vi "Dashboard Main.vi"() -> ()   [LabVIEW 2018]
uses:
  <vilib>/Utility/miscctls.llb/LVBoundsTypeDef.ctl
  <vilib>/Utility/miscctls.llb/LVRowAndColumnTypeDef.ctl
  <vilib>/event_ctls.llb/eventvkey.ctl
  <vilib>/Rock Robotics/Network Tables/NT Read Numeric Array.vi
  <vilib>/Rock Robotics/Network Tables/NT Write Boolean.vi
  <vilib>/Rock Robotics/WPI/Dashboard/WPI_DashboardLogging Global.vi
panel:
  in  "Camera Settings Right":T1={"Frame Rate"=30, "Compression"=30, "Size"=1, "DB Camera Config"=FALSE} {"Frame Rate" scale=1.0..30.0; "Compression" scale=100.0..-1.0; "Size" items=["640x480", "320x240", "160x120"]}
  in  "Camera Name Right":string(combo)="No Camera Selection"
  out "Camera Perf":string
  in  "Camera Settings":T1={"Frame Rate"=30, "Compression"=30, "Size"=1, "DB Camera Config"=FALSE} {"Frame Rate" scale=1.0..30.0; "Compression" scale=100.0..-1.0; "Size" items=["640x480", "320x240", "160x120"]}
  in  "TCP":refnum<k5>
  in  "Rec Mode":enum32{"Stop", "Record", "Playback"}(radio)
  out "Robot IP":string
  out "Image Message":string="Timeout in Camera Communications"
  in  "Dashboard Tab":T2(tab)
  in  "Select Auto":string(combo)="Select Autonomous ..."
  out "NT Connection":bool
  out "MotorChart R":cluster{"Numeric":dbl, "Numeric":dbl}(graph)
  out "MotorChart L":cluster{"Numeric":dbl, "Numeric":dbl}(graph)
  out "MotorSliders R":cluster{"MotorSlide1":dbl, "MotorSlide2":dbl} {"MotorSlide2" scale=-1.0..1.0 scale format="%#_2e"; "MotorSlide1" scale=-1.0..1.0 scale format="%#_2e"}
  out "MotorSliders L":cluster{"MotorSlide1":dbl, "MotorSlide2":dbl} {"MotorSlide2" scale=-1.0..1.0 scale format="%#_2e"; "MotorSlide1" scale=-1.0..1.0 scale format="%#_2e"}
  out "Gyro_defualt":dbl(knob) scale=0.0..360.0
  out "JS1 Z":dbl(slide) scale=-1.0..1.0 scale format="%#_2e"
  out "JS1 Graph":cluster{"X":dbl, "Y":dbl}[](graph)
  out "JS1 Buttons":T3
  out "JS2 Z":dbl(slide) scale=-1.0..1.0 scale format="%#_2e"
  out "JS2 Graph":cluster{"X":dbl, "Y":dbl}[](graph)
  out "JS2 Buttons":T3
  out "Mode":T4(ring)=enum."Auto Disabled"
  out "Right Camera Perf":cluster{"Bandwidth (Mbps)":dbl, "FPS":dbl}
  out "Camera Image Right":T5(plugin-control)
  in  "DB/String 9":string
  in  "DB/String 8":string
  in  "DB/String 7":string
  in  "DB/String 6":string
  in  "DB/String 5":string
  in  "DB/String 4":string
  in  "DB/String 3":string
  in  "DB/String 2":string
  in  "DB/String 1":string
  in  "DB/String 0":string
  in  "DB/Slider 0":dbl(slide) scale=0.0..5.0
  in  "DB/Slider 1":dbl(slide) scale=0.0..5.0
  in  "DB/Slider 2":dbl(slide) scale=0.0..5.0
  in  "DB/Slider 3":dbl(slide) scale=0.0..5.0
  out "DB/LED 3":bool
  out "DB/LED 2":bool
  out "DB/LED 1":bool
  out "DB/LED 0":bool
  in  "DB/Button 3":bool
  in  "DB/Button 2":bool
  in  "DB/Button 1":bool
  in  "DB/Button 0":bool caption="New Name"
  out "Gyro":dbl
  out "Cargo 0":bool
  out "Cargo 3":bool
  out "Cargo 1":bool
  out "Cargo 2":bool
  out "Hatch 2":bool
  out "Hatch 0":bool
  out "Hatch 1":bool
  out "Elevator Position":dbl(slide) scale=0.0..20000.0
  out "Cargo Drop":bool
  out "Cargo Pick Up":bool
  out "Carry":bool
  out "Hatch":bool
  in  "Calibrate?":bool
  out "PickUp/DropOff":string
  out "SwerveMode":string
  in  "Test Slider":dbl(slide) scale=0.0..100.0 scale format="%#_3g"
  in  "On/Off":bool caption="Solenoid"
  in  "Test Name":u16(ring) items=["Select the test to run..."]
  in  "Test Tree":string(tree)
  in  "Motor":cluster{"Value":dbl, "Enable":bool} {"Value" scale=-1.0..1.0 scale format="%#_3g"}
  out "Progress":T6 {"Test Progress" scale=0.0..100.0}
  in  "Rev/Fwd":cluster{"Forward":bool, "Reverse":bool}
  in  "Test Ring":u16(ring) items=["Monochrome", "Color"]
  out "Cmd Status":string
  in  "Execute Command":bool
  in  "Command Params":string[][](table)
  in  "Command Selection":i32(listbox)
  in  "CheckList":i32(listbox)
  out "Tree":string(tree)
  out "Camera Image":T5(plugin-control)
  out "Background":bool
  in  "Camera Name":string(combo)="No Camera Selection"
  # "HW"
  # "HW"
  # "Joysticks"
  # "Drive Motors"
  # "Front"
  # "Right"
  # "Left"
  # "Back"
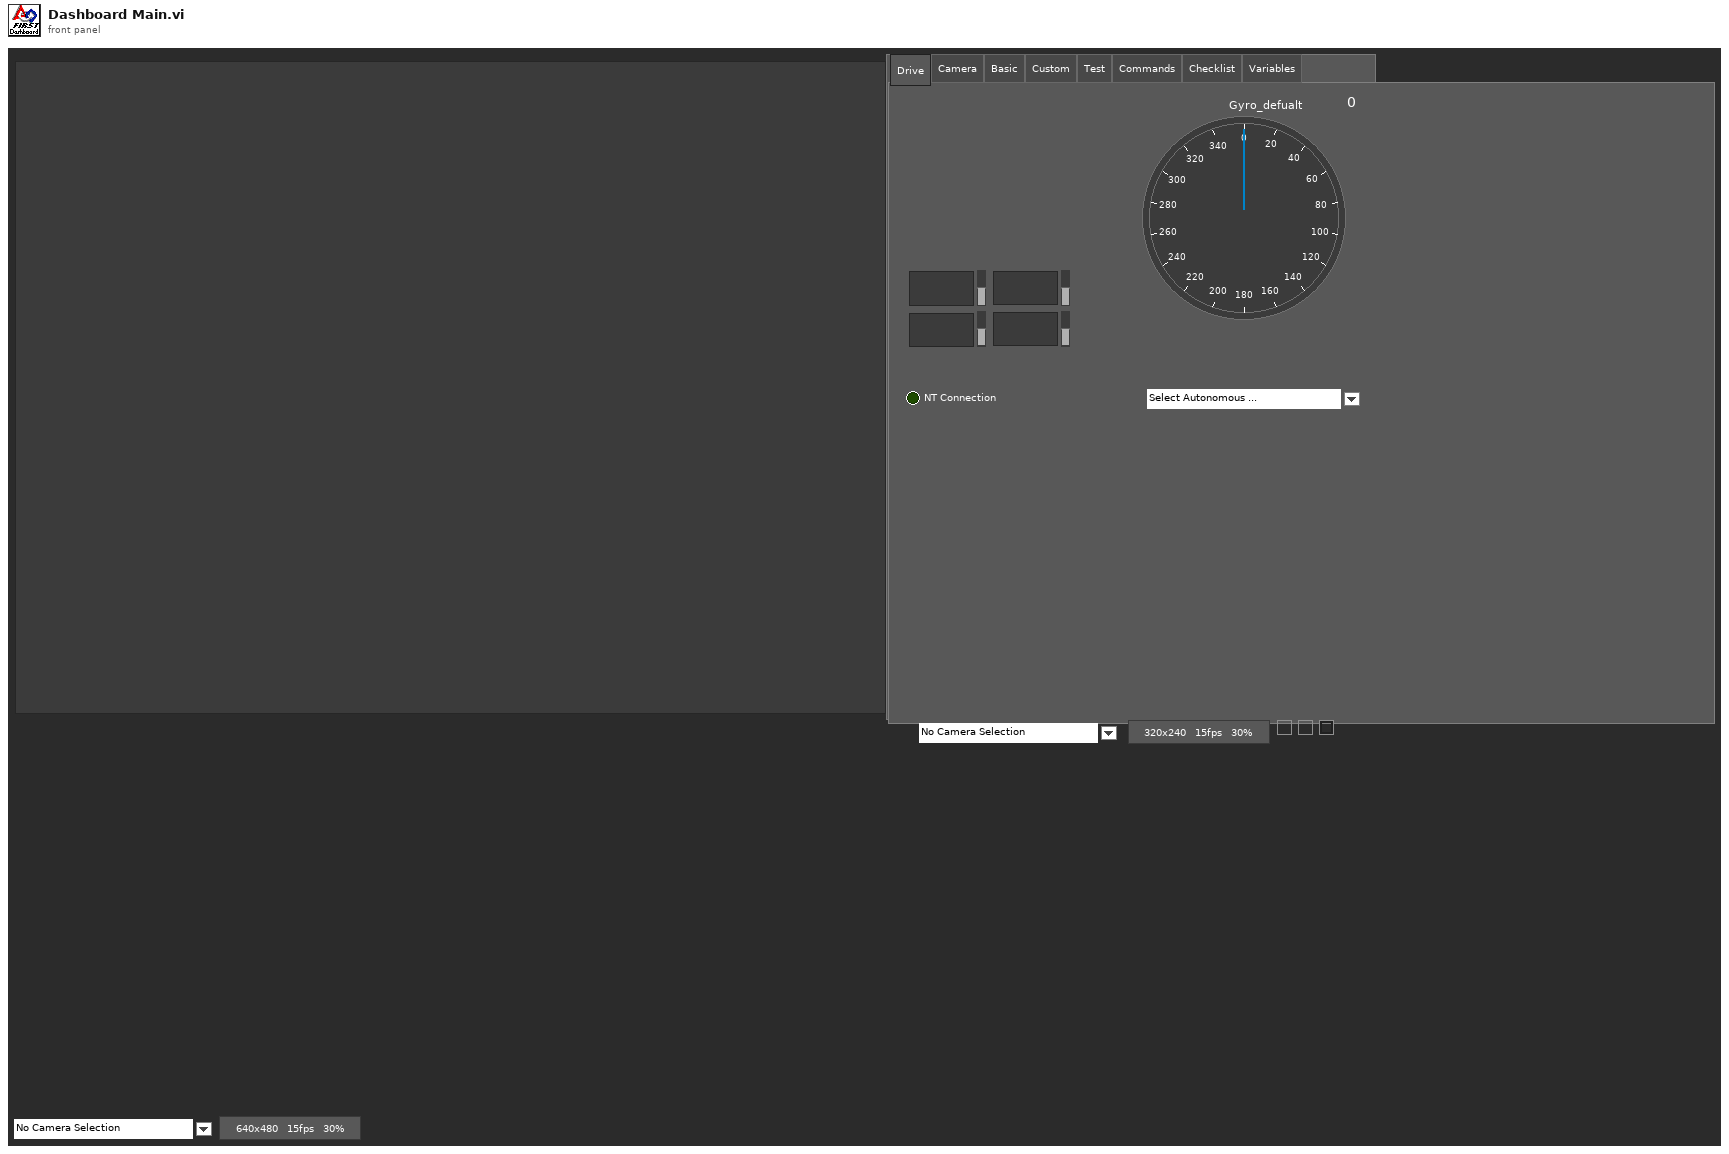
[diagram p1: front panel]
types:
  T1 = cluster{"Frame Rate":i32, "Compression":i32, "Size":u16, "DB Camera Config":bool}
  T2 = enum32{"Drive", "Camera", "Basic", "Custom", "Test", "Commands", "Checklist", "Variables"}
  T3 = cluster{bool, bool, bool, bool, bool, bool, bool, bool, bool, bool, bool, bool}
  T4 = enum8{"Tele-Op Disabled", "Tele-Op Enabled", "Auto Disabled", "Auto Enabled", "Test Disabled", "Test Enabled", "Disconnected", "No Code", "E-Stop"}
  T5 = typedef "IMAQ Image.ctl" = refnum<image>
  T6 = cluster{"Test Progress":u8, "Test Progress Text":string}
  T7 = typedef "LVBoundsTypeDef.ctl" = cluster{"Width":u32, "Height":u32}
  T8 = cluster{"Save Path":path, "Interval (s)":dbl, "Keep":i32}
  T9 = typedef "Image Type" = u32
  T10 = cluster{"IDs":cluster{"RPC field ID":u16, "Unique ID":u16}, "String":string}
  T11 = cluster{"Error Strings":string, "Disable Counts":cluster{u16, u16}, "Rail Faults":cluster{u16, u16, u16}, "Robot IP":string, "DB Mode":u8, "Event Info":cluster{"Name":string, "Type":u8, "Number":u16, "Replay":u8}}
  T12 = cluster{"Storage":cluster{"Disk Free":u64, "RAM Block":u32, "RAM free":u32}, "CPU Utilization":cluster{"CPU % ISR":sgl, "CPU % Time Crit":sgl, "CPU % Timed Str":sgl, "CPU % High":sgl, "CPU % Above":sgl, "CPU % Normal":sgl, "CPU % Low":sgl}, "CAN":cluster{"% Bus Utilization":sgl, "Bus Off Cnt":u32, "TX_FIFO Full Cnt":u32, "Receive Error Cnt":u8, "Transmit Error Cnt":u8}, "HID":cluster{"HID Outputs":u32, "Rumble Low":u16, "Rumble High":u16}[]}
  T13 = cluster{"Status bits":cluster{"Test Mode":bool, "Autonomous":bool, "Enabled":bool, "Code Start":bool, "Brownout":bool, "Reserved 2":bool, "Reserved 3":bool, "E-Stop":bool}, "Code Trace":cluster{"Disabled":bool, "TeleOp":bool, "Auto":bool, "Test":bool}, "Controller Type":enum16{"unknown", "cRIO", "roboRio"}, "Code?":enum16{"unknown", "noCode", "code"}, "Battery V":dbl}
  T14 = cluster{"Control Bits":cluster{"TestMode":bool, "Autonomous":bool, "Enabled":bool, "FMS Present":bool, bool, bool, bool, "E-Stop":bool}, "Team Station ":u8, "Countdown":sgl, "Joystick Values":cluster{"Axes":dbl[], "Buttons":bool[], "POVs":i16[]}[]}
  T15 = cluster{"Axes":dbl[], "Buttons":bool[], "POVs":i16[]}[]
  T16 = cluster{"Axes":dbl[], "Buttons":bool[], "POVs":i16[]}
  T17 = cluster{"Buttons[0]":bool, "Buttons[1]":bool, "Buttons[2]":bool, "Buttons[3]":bool, "Buttons[4]":bool, "Buttons[5]":bool, "Buttons[6]":bool, "Buttons[7]":bool, "Buttons[8]":bool, "Buttons[9]":bool, "Buttons[10]":bool, "Buttons[11]":bool}
  T18 = cluster{"Camera Image":refnum<vi>, "Dashboard Tab":refnum<vi>, "Background":refnum<vi>, "Rec Mode":refnum<vi>, "Test Slider":refnum<vi>, "On/Off ":refnum<vi>, "Test Ring":refnum<vi>, "Rev/Fwd":refnum<vi>, "Test Name":refnum<vi>, "Motor":refnum<vi>, "Progress":refnum<vi>, "CheckList":refnum<vi>, "Tree":refnum<vi>, "Test Tree":refnum<vi>, "Command Params":refnum<vi>, "Command Selection":refnum<vi>, "Execute Command":refnum<vi>, "Cmd Status":refnum<vi>, "Camera Settings":refnum<vi>, "Camera Name":refnum<vi>, "Camera Perf":refnum<vi>, "Camera Settings Right":refnum<vi>, "Camera Name Right":refnum<vi>, "Camera Image Right":refnum<vi>}
  T19 = cluster{"Global Rectangle":i32[], "Contours":cluster{"Contour Type":u32, "ROI Type":u32, "Points":i32[]}[]}
  T20 = cluster{"Camera Name":string, string, "Saved DB Images Info":cluster{"Save Path":path, "Interval (s)":dbl, "Keep":i32}}
  T21 = cluster{"Camera Name Right":string, string, "Saved DB Images Info":cluster{"Save Path":path, "Interval (s)":dbl, "Keep":i32}}
  T22 = cluster{"Operation":enum16{"Update", "Clear"}, "Color Box":u32}[]
  T23 = typedef "eventvkey.ctl" = enum16{"ASCII", "Enter", "Return", "Shift", "Ctrl", "Alt", "Cmd", "Opt", "Caps", "NumLock", "Clear", "Break", "Up", "Down", "Left", "Right", "Insert", "Delete", "Home", "End", "PageUp", "PageDown", "Escape", "Help", "Pause", "ScrollLock", "F1", "F2", "F3", "F4", "F5", "F6", "F7", "F8", "F9", "F10", "F11", "F12", "F13", "F14", "F15", "F16", "F17", "F18", "F19", "F20", "F21", "F22", "F23", "F24", "Play", "VolumeUp", "VolumeDown", "Mute", "Two Byte Char"}
  T24 = cluster{"Image Size":bool, "Image Type":bool, "Pixel Value":bool, "ROI Information":bool, "Zoom Factor":bool}
  T25 = cluster{"Operation":enum16{"Update", "Clear"}, "Color Box":u32}
  T26 = typedef "LVRowAndColumnTypeDef.ctl" = cluster{"Row":i32, "Column":i32}
  T27 = cluster{"Shift":bool, "Ctrl":bool, "Alt":bool, "Cmd":bool, "Opt":bool}
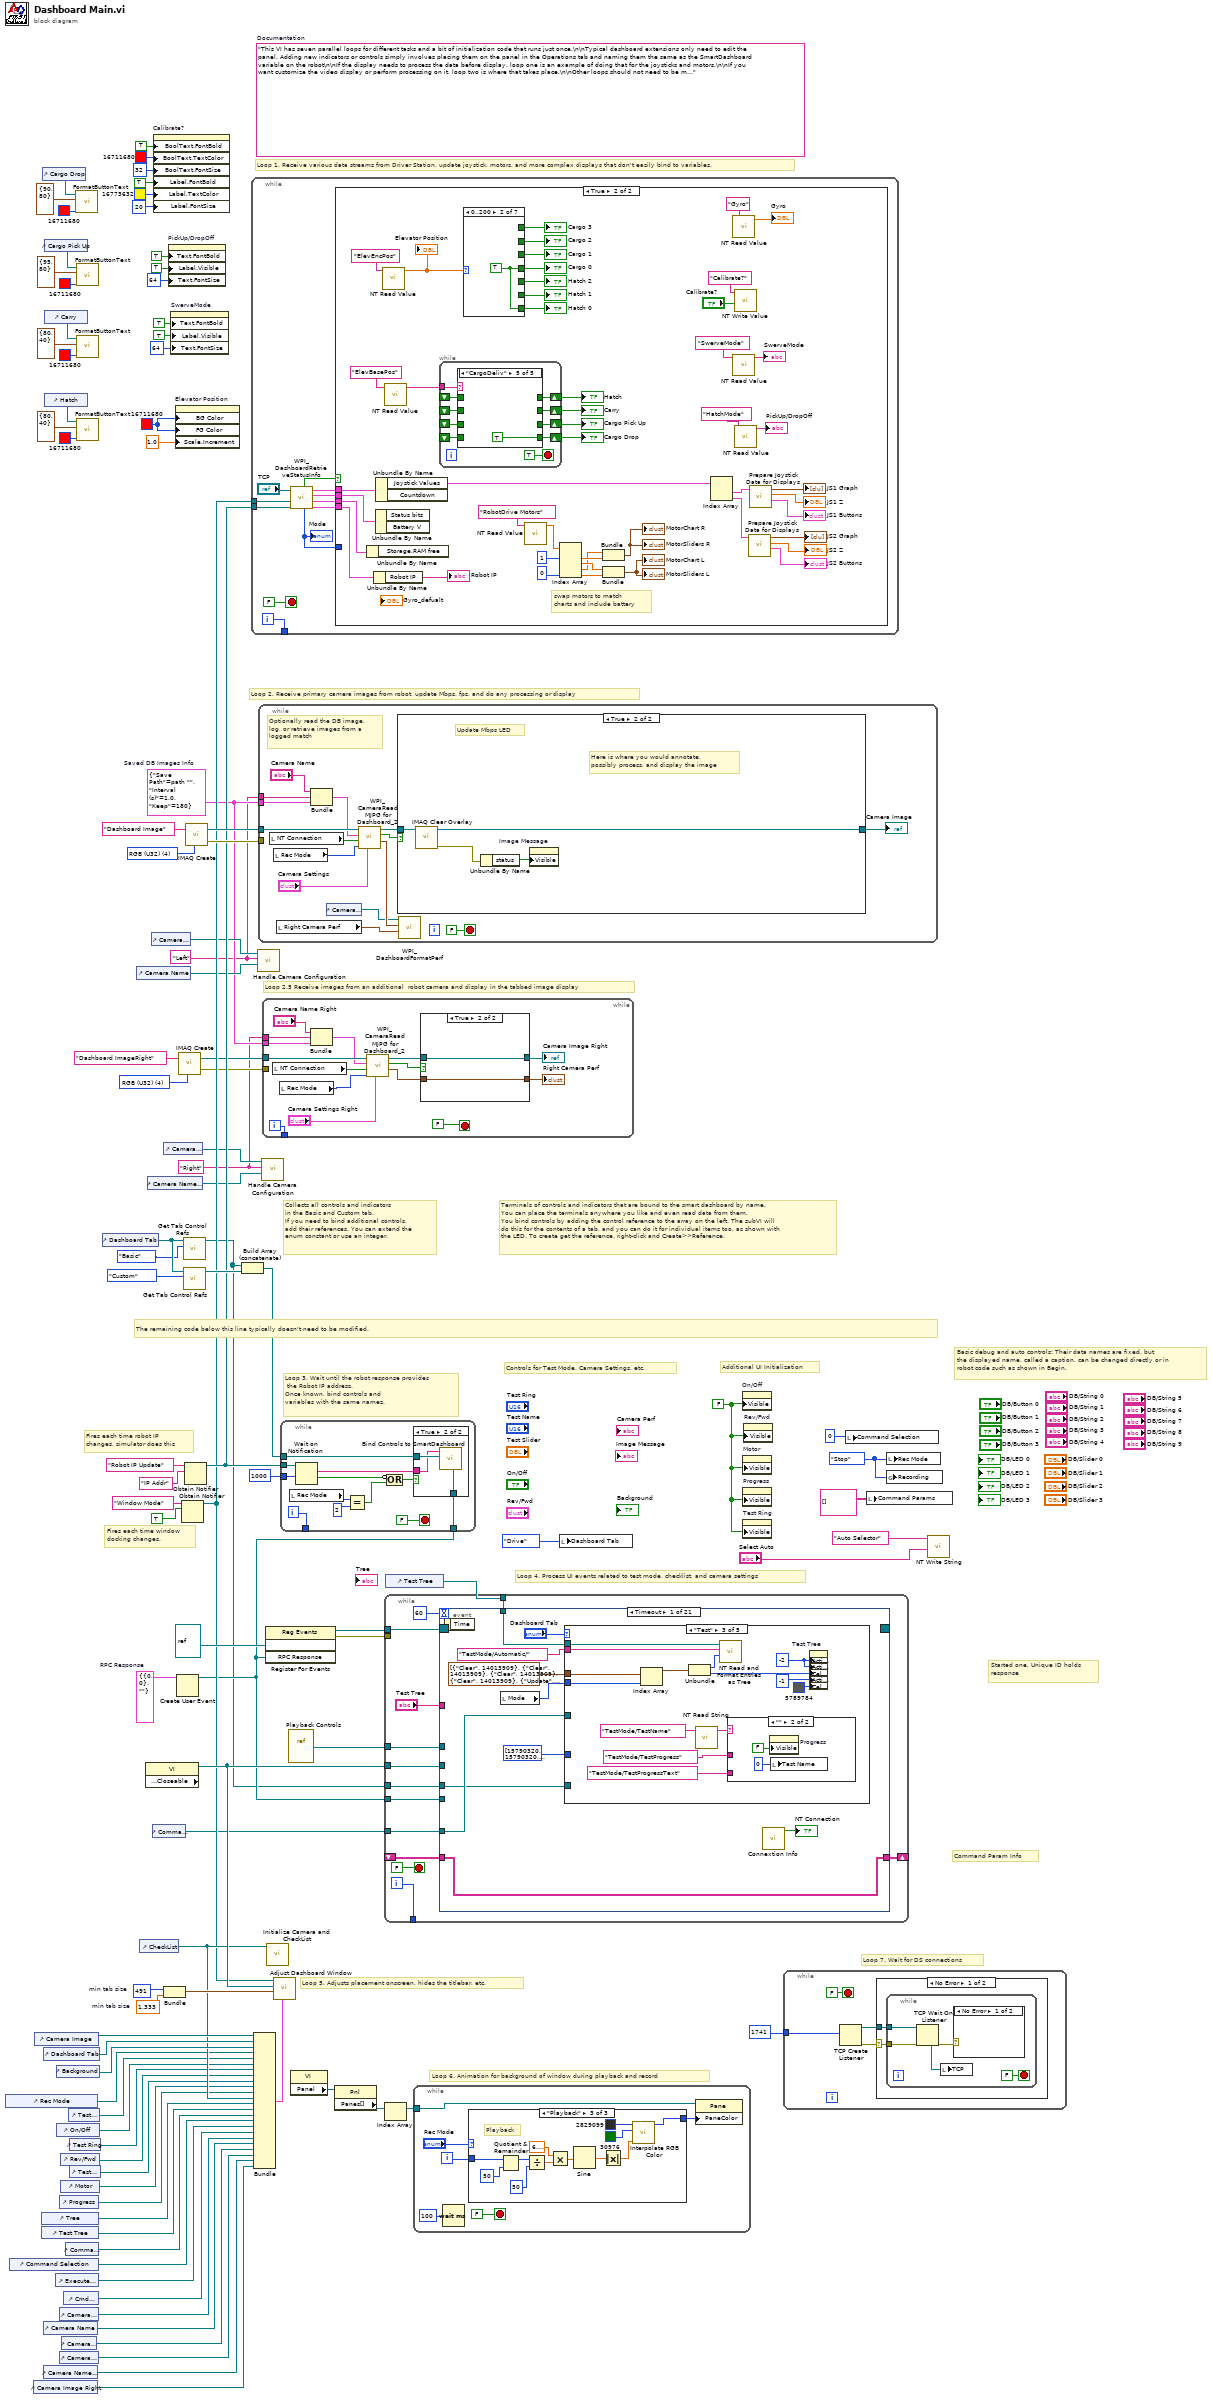
[diagram p0: block diagram]
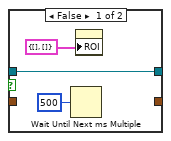
[diagram p2: hidden frame]
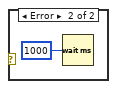
[diagram p3: hidden frame]
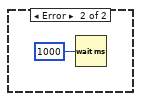
[diagram p4: hidden frame]
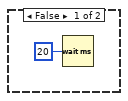
[diagram p5: hidden frame]
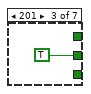
[diagram p7: hidden frame]
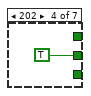
[diagram p8: hidden frame]
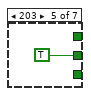
[diagram p9: hidden frame]
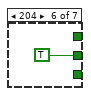
[diagram p10: hidden frame]
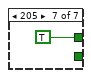
[diagram p11: hidden frame]
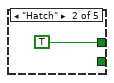
[diagram p13: hidden frame]
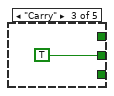
[diagram p14: hidden frame]
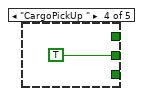
[diagram p15: hidden frame]
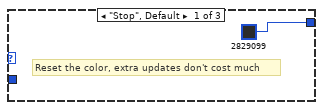
[diagram p16: hidden frame]
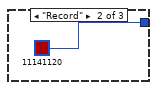
[diagram p17: hidden frame]
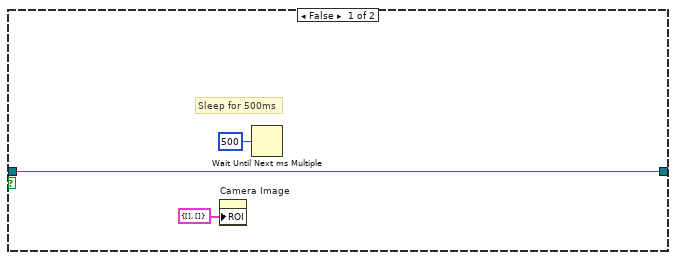
[diagram p19: hidden frame]
diagram:
  w2 = u32 16711680
  w29 = T8 {"Save Path"=path "", "Interval (s)"=1.0, "Keep"=180}  # Saved DB Images Info
  w28 = "Right"
  w27 = "Left"
  w39 = T9 4 items=["Grayscale (U8)", "Grayscale (I16)", "Grayscale (SGL)", "Complex (CSG)", "RGB (U32)", "HSL (U32)", "RGB (U64)"] ("Image Type")
  w55 = T10 {"IDs"={"RPC field ID"=0, "Unique ID"=0}, "String"=""}  # RPC Response
  w78 = 491  # min tab size
  w77 = 1.333  # min tab size
  w85 = enum32{"Stop", "Record", "Playback"}."Stop" ("Rec Mode")
  w62 = FALSE ("Visible")
  (unwired) "This VI has seven parallel loops for different tasks and a bit of initialization code that runs just once.\n\nTypical dashboard extensions only need to edit the panel. Adding new indicators or controls simply involves placing them on the panel in the Operations tab and naming them the same as the SmartDashboard variable on the robot\n\nIf the display needs to process the data before display, loop one is an example of doing that for the joysticks and motors.\n\nIf you want customize the video display or perform processing on it, loop two is where that takes place.\n\nOther loops should not need to be modified. They are pretty standard, and document the task they perform."  # Documentation
  w102 = T9 4 items=["Grayscale (U8)", "Grayscale (I16)", "Grayscale (SGL)", "Complex (CSG)", "RGB (U32)", "HSL (U32)", "RGB (U64)"] ("Image Type")
  # "Loop 2.5 Receive images from an additional  robot camera and display in the tabbed image display"
  # "Command Param Info"
  # "Started one, Unique ID holds\nresponse"
  # "Loop 7. Wait for DS connections"
  # "Basic debug and auto controls: Their data names are fixed, but\nthe displayed name, called a caption, can be changed directly or in\nrobot code such as shown in Begin."
  # "Controls for Test Mode, Camera Settings, etc."
  # "Additional UI Initialization"
  # "Loop 6. Animation for background of window during playback and record"
  # "Fires each time robot IP\nchanges, simulator does this"
  # "Fires each time window\ndocking changes."
  # "Collects all controls and indicators\nin the Basic and Custom tab.\nIf you need to bind additional controls,\nadd their references. You can extend the\nenum constant or use an integer."
  # "The remaining code below this line typically doesn't need to be modified."
  # "Loop 4. Process UI events related to test mode, checklist, and camera settings"
  # "Terminals of controls and indicators that are bound to the smart dashboard by name.\nYou can place the terminals anywhere you like and even read data from them.\nYou bind controls by adding the control reference to the array on the left. The subVI will\ndo this for the contents of a tab, and you can do it for individual items too, as shown with\nthe LED. To create get the reference, right-click and Create>>Reference."
  # "Loop 3. Wait until the robot response provides\n the Robot IP address.\nOnce known, bind controls and\nvariables with the same names."
  # "Loop 5. Adjusts placement onscreen, hides the titlebar, etc."
  # "Loop 1. Receive various data streams from Driver Station, update joystick, motors, and more complex displays that don't easily bind to variables."
  # "Loop 2. Receive primary camera images from robot, update Mbps, fps, and do any processing or display"
  n1 = control-ref of="Rec Mode"() -> (w68:refnum<vi>)
  n2 = control-ref of="Command Selection"() -> (w54:refnum<vi>)
  n3 = control-ref of="Camera Image Right"() -> (w32:refnum<vi>)
  n4 = control-ref of="Camera Image"() -> (w80:refnum<vi>)
  n5 = control-ref of="Tree"() -> (w72:refnum<vi>)
  n6 = control-ref of="Test Tree"() -> (w71:refnum<vi>)
  n7 = control-ref of="Cargo Drop"() -> (w14:refnum<vi>)
  n8 = control-ref of="Dashboard Tab"() -> (w79:refnum<vi>)
  n9 = control-ref of="Camera Name"() -> (w45:refnum<vi>)
  n10 = control-ref of="Camera Name Right"() -> (w33:refnum<vi>)
  n11 = control-ref of="Cargo Pick Up"() -> (w9:refnum<vi>)
  n12 = control-ref of="Carry"() -> (w8:refnum<vi>)
  n13 = control-ref of="Hatch"() -> (w3:refnum<vi>)
  n14 = control-ref of="Execute Command"() -> (w56:refnum<vi>)
  n15 = control-ref of="Background"() -> (w75:refnum<vi>)
  n16 = control-ref of="On/Off"() -> (w66:refnum<vi>)
  n17 = control-ref of="Progress"() -> (w63:refnum<vi>)
  n18 = control-ref of="Camera Settings"() -> (w46:refnum<vi>)
  n19 = control-ref of="Camera Settings Right"() -> (w34:refnum<vi>)
  n20 = control-ref of="Rev/Fwd"() -> (w64:refnum<vi>)
  n21 = control-ref of="Motor"() -> (w69:refnum<vi>)
  n22 = control-ref of="Camera Perf"() -> (w44:refnum<vi>)
  n23 = control-ref of="Cmd Status"() -> (w50:refnum<vi>)
  n24 = control-ref of="Command Params"() -> (w57:refnum<vi>)
  n25 = control-ref of="Test Slider"() -> (w67:refnum<vi>)
  n26 = control-ref of="Test Ring"() -> (w65:refnum<vi>)
  n27 = control-ref of="Test Name"() -> (w70:refnum<vi>)
  n28 = call "FormatButtonText.vi"("TextColor"=u32 16711680, "TextBoxSize"=T7 {"Width"=90, "Height"=80} ("Boolean Text.Size 2"), "Button"=w14) -> ()  [unwired: 9 in]
  n29 = call "FormatButtonText.vi"("TextColor"=u32 16711680, "TextBoxSize"=T7 {"Width"=95, "Height"=80} ("Boolean Text.Size 2"), "Button"=w9) -> ()  [unwired: 9 in]
  n30 = call "FormatButtonText.vi"("TextColor"=u32 16711680, "TextBoxSize"=T7 {"Width"=80, "Height"=40} ("Boolean Text.Size 2"), "Button"=w8) -> ()  [unwired: 9 in]
  n31 = call "FormatButtonText.vi"("TextColor"=u32 16711680, "TextBoxSize"=T7 {"Width"=80, "Height"=40} ("Boolean Text.Size 2"), "Button"=w3) -> ()  [unwired: 9 in]
  n32 = control-ref of="Dashboard Tab"() -> (w83:refnum<vi>)
  n33 = control-ref of="Camera Name"() -> (w47:refnum<vi>)
  n34 = control-ref of="CheckList"() -> (w73:refnum<vi>)
  n35 = property class="VI" props=["Front Panel.Closeable"]() -> (reference out=w84:refnum<vi>)  [unwired: 2 in, 2 out]
  n36 = control-ref of="Camera Name Right"() -> (w35:refnum<vi>)
  n37 = control-ref of="Camera Settings"() -> (w48:refnum<vi>)
  n38 = control-ref of="Command Params"() -> (w49:refnum<vi>)
  n39 = property on="Calibrate?" class="Bool (strict)"("BoolText.FontBold"=TRUE ("Boolean Text.Font:Bold"), "BoolText.TextColor"=u32 16711680, "BoolText.FontSize"=u32 32 ("Boolean Text.Font:Size"), "Label.FontBold"=TRUE ("Boolean Text.Font:Bold"), "Label.TextColor"=u32 16773632, "Label.FontSize"=u32 20 ("Boolean Text.Font:Size")) -> ()  [unwired: 2 in, 2 out]
  n40 = control-ref of="Camera Settings Right"() -> (w36:refnum<vi>)
  n41 = Bundle("min tab size"=w78, "min tab size"=w77) -> (w76:cluster{"min tab size":i32, "min tab size":dbl})  [unwired: 1 in]
  n42 = property on="PickUp/DropOff" class="Str"("Text.FontBold"=TRUE ("Text.Font:Bold"), "Label.Visible"=TRUE, "Text.FontSize"=u32 64 ("Text.Font:Size")) -> ()  [unwired: 2 in, 2 out]
  n43 = property on="SwerveMode" class="Str"("Text.FontBold"=TRUE ("Text.Font:Bold"), "Label.Visible"=TRUE, "Text.FontSize"=u32 64 ("Text.Font:Size")) -> ()  [unwired: 2 in, 2 out]
  n44 = property on="Elevator Position" class="Slide (strict)"("BG Color"=w2, "FG Color"=w2, "Scale.Increment"=1.0 ("Scale.Range:Increment")) -> ()  [unwired: 2 in, 2 out]
  n45 = Create User Event(user event datatype=w55) -> (user event=w51:refnum<user-event>)  [unwired: 1 in, 1 out]
  n46 = call "IMAQ Create"("Image Name"="Dashboard ImageRight", "Image Type"=w39) -> ("New Image"=w38:T5, "error out"=w37:errorcluster)  [unwired: 2 in, 1 out]
  n47 = Obtain Notifier(name (unnamed)="Window Mode", notification data type=TRUE) -> (notifier out=w60:refnum<notifier>)  [unwired: 2 in, 2 out]
  n48 = call <vilib>:"Get Tab Control Refs.vi"("Page Index"=T2."Basic" ("Dashboard Tab"), "TabControl in"=w83) -> ("ControlsOnPage"=w43:refnum<vi>[])  [unwired: 9 in]
  n49 = call <vilib>:"Get Tab Control Refs.vi"("Page Index"=T2."Custom" ("Dashboard Tab"), "TabControl in"=w83) -> ("ControlsOnPage"=w82:refnum<vi>[])  [unwired: 9 in]
  n50 = Obtain Notifier(name (unnamed)="Robot IP Update", notification data type="IP Addr" ("name (unnamed)")) -> (notifier out=w61:refnum<notifier>)  [unwired: 2 in, 2 out]
  n51 = call "IMAQ Create"("Image Name"="Dashboard Image", "Image Type"=w102) -> ("New Image"=w100:T5, "error out"=w99:errorcluster)  [unwired: 2 in, 1 out]
  n52 = Build Array (concatenate)(w43, w82) -> (w81:refnum<vi>[])
  n53 = while {
    tunnel: [w112] -> _
    tunnel: w61 -> [w107]
    tunnel: w60 -> [w104]
    i -> [w112]
    stop <- FALSE stop-if-true
    n54 = call <vilib>:"WPI_DashboardRetrieveStatusInfo.vi"("Binding Refnum"=w107, "Window Mode Notifier"=w104, "TCP Cnx"="TCP") -> ("Power and Errors"=w108:T11, "Robot Metrics"=w110:T12, "Status Info"=w111:T13, "Control Info"=w109:T14, "Robot Mode"=w106:T4, "Process?"=w103:bool)  [unwired: 3 in]
    "Mode" <- w106
    n55 = case shown="True" w103 {
      tunnel: w111 -> [_ w161]
      tunnel: w110 -> [_ w160]
      tunnel: w109 -> [_ w159]
      tunnel: w108 -> [_ w158]
      tunnel: w106 -> [_ _]
      frame False {
        n56 = Wait (ms)(milliseconds to wait=u32 20) -> ()  [unwired: 1 out]
      }
      frame True {
        # "swap motors to match\ncharts and include battery"
        n57 = Unbundle By Name(w160) -> ()  [unwired: 1 out]
        n58 = Unbundle By Name(w158) -> ("Robot IP"=→"Robot IP":string)
        n59 = Unbundle By Name(w161) -> ()  [unwired: 2 out]
        n60 = Unbundle By Name(w159) -> ("Joystick Values"=w149:T15)  [unwired: 1 out]
        n61 = call-poly <vilib>:"NT Read Value.vi"("Name"="ElevEncPos") -> ("Numeric"=w124:dbl)  [unwired: 9 in, 1 out]
        "Elevator Position" <- w124
        n62 = call-poly <vilib>:"NT Read Value.vi"("Name"="ElevBasePos") -> ("String"=w129:string)  [unwired: 9 in, 1 out]
        n63 = while {
          tunnel: w129 -> [w177]
          shift-right: [w175] -> w127
          shift-left: _ -> [w171]
          shift-right: [w173] -> w126
          shift-left: _ -> [w170]
          shift-right: [w174] -> w125
          shift-left: _ -> [w169]
          shift-right: [w176] -> w128
          shift-left: _ -> [w168]
          stop <- TRUE stop-if-true
          n64 = case shown="\"CargoDeliv\"" w177 {
            tunnel: [w178 _ _ _ TRUE ("Cargo Pick Up")] -> w176
            tunnel: [w181 TRUE ("Hatch") _ _ _] -> w175
            tunnel: [w179 _ _ TRUE ("Cargo Pick Up") _] -> w174
            tunnel: [w180 _ TRUE ("Cargo Pick Up") _ _] -> w173
            tunnel: w171 -> [w181 _ _ _ _]
            tunnel: w170 -> [w180 _ _ _ _]
            tunnel: w169 -> [w179 _ _ _ _]
            tunnel: w168 -> [w178 _ _ _ _]
            frame "No Change", Default {
            }
            frame "Hatch" {
            }
            frame "Carry" {
            }
            frame "CargoPickUp " {
            }
            frame "CargoDeliv" {
            }
          }
        }
        "Hatch" <- w127
        "Carry" <- w126
        "Cargo Pick Up" <- w125
        "Cargo Drop" <- w128
        n65 = case shown="0..200" w124 {
          tunnel: [_ _ _ _ _ _ TRUE] -> w123
          tunnel: [_ _ _ _ _ TRUE _] -> w122
          tunnel: [_ _ _ _ TRUE _ _] -> w121
          tunnel: [_ w162 _ _ _ _ _] -> w120
          tunnel: [_ _ _ TRUE _ _ _] -> w119
          tunnel: [_ _ TRUE _ _ _ _] -> w118
          tunnel: [_ w162 _ _ _ _ _] -> w117
          frame -1, Default {
          }
          frame 0..200 {
            w162 = TRUE
          }
          frame 201 {
          }
          frame 202 {
          }
          frame 203 {
          }
          frame 204 {
          }
          frame 205 {
          }
        }
        "Hatch 1" <- w118
        "Hatch 0" <- w117
        "Hatch 2" <- w119
        "Cargo 2" <- w122
        "Cargo 1" <- w121
        "Cargo 3" <- w123
        "Cargo 0" <- w120
        n66 = call-poly <vilib>:"NT Read Value.vi"("Name"="RobotDrive Motors") -> ("Numeric Array"=w139:dbl[])  [unwired: 9 in, 1 out]
        n67 = Index Array(array=w139, index #1=1, index #4=0) -> (element #1=w153:dbl, element #2=w154:dbl, element #3=w152:dbl, element #4=w157:dbl)  [unwired: 2 in]
        n68 = Bundle("Numeric"=w152, "Numeric"=w153) -> (→"MotorChart R" →"MotorSliders R":cluster{"Numeric":dbl, "Numeric":dbl})  [unwired: 1 in]
        n69 = Bundle("Numeric"=w154, "Numeric"=w157) -> (→"MotorChart L" →"MotorSliders L":cluster{"Numeric":dbl, "Numeric":dbl})  [unwired: 1 in]
        n70 = Index Array(array=w149) -> (element #1=w148:T16, element #2=w144:T16)  [unwired: 2 in]
        n71 = call-poly <vilib>:"NT Read Value.vi"("Name"="Gyro") -> ("Numeric"=→"Gyro":dbl)  [unwired: 9 in, 1 out]
        n72 = call-poly <vilib>:"NT Read Value.vi"("Name"="SwerveMode") -> ("String"=→"SwerveMode":string)  [unwired: 9 in, 1 out]
        n73 = call-poly <vilib>:"NT Write Value.vi"("Boolean"="Calibrate?", "Name"="Calibrate?") -> ()  [unwired: 9 in, 1 out]
        n74 = call-poly <vilib>:"NT Read Value.vi"("Name"="HatchMode") -> ("String"=→"PickUp/DropOff":string)  [unwired: 9 in, 1 out]
        n75 = call "Prepare Joystick Data for Displays.vi"("Joystick Values"=w144) -> ("Buttons"=→"JS2 Buttons":T17, "Z Axis"=→"JS2 Z":dbl, "Cartesian Data"=→"JS2 Graph":cluster{"X axis":dbl, "X axis":dbl}[])  [unwired: 8 in]
        n76 = call "Prepare Joystick Data for Displays.vi"("Joystick Values"=w148) -> ("Buttons"=→"JS1 Buttons":T17, "Z Axis"=→"JS1 Z":dbl, "Cartesian Data"=→"JS1 Graph":cluster{"X axis":dbl, "X axis":dbl}[])  [unwired: 8 in]
      }
    }
  }
  n77 = Bundle("Camera Image"=w80, "Dashboard Tab"=w79, "Background"=w75, "Rec Mode"=w68, "Test Slider"=w67, "On/Off"=w66, "Test Ring"=w65, "Rev/Fwd"=w64, "Test Name"=w70, "Motor"=w69, "Progress"=w63, "CheckList"=w73, "Tree"=w72, "Test Tree"=w71, "Command Params"=w57, "Command Selection"=w54, "Execute Command"=w56, "Cmd Status"=w50, "Camera Settings"=w46, "Camera Name"=w45, "Camera Perf"=w44, "Camera Settings Right"=w34, "Camera Name Right"=w33, "Camera Image Right"=w32) -> (w74:T18)  [unwired: 1 in]
  n78 = call "Handle Camera Configuration.vi"("CameraNameRef"=w47, "Display Name"=w27, "ClusterRef"=w48) -> ()  [unwired: 9 in]
  n79 = while {
    tunnel: w100 -> [w199]
    tunnel: w99 -> [_]
    tunnel: w29 -> [w192]
    tunnel: w27 -> [w189]
    stop <- FALSE stop-if-true
    # "Optionally read the DB image,\nlog, or retrieve images from a\nlogged match"
    n80 = local read "NT Connection"() -> (w193:bool)
    n81 = local read "Rec Mode"() -> (w196:enum32{"Stop", "Record", "Playback"})
    n82 = local read "Right Camera Perf"() -> (w187:cluster{"Bandwidth (Mbps)":dbl, "FPS":dbl})
    n83 = Bundle("Camera Name"="Camera Name", w189, "Saved DB Images Info"=w192) -> (w191:T20)  [unwired: 1 in]
    n84 = control-ref of="Camera Perf"() -> (w186:refnum<vi>)
    n85 = call <vilib>:"WPI_CameraRead MJPG for Dashboard_2.vi"("Camera Settings"="Camera Settings", "Rec Mode"=w196, "NT Connection"=w193, "Capture Info"=w191, "Image in"=w199) -> ("perf info"=w188:cluster{"Bandwidth (Mbps)":dbl, "fps":dbl}, "Active"=w197:bool, "Image\\ out"=w198:T5)  [unwired: 4 in]
    n86 = case shown="True" w197 {
      tunnel: w198 -> [w202 w205]
      tunnel: [w202 w204] -> w194
      frame False {
        # "Sleep for 500ms"
        n87 = property on="Camera Image" class="ImageControl"("ROI"=T19 {"Global Rectangle"=[], "Contours"=[]}) -> ()  [unwired: 2 in, 2 out]
        n88 = Wait Until Next ms Multiple(millisecond multiple=u32 500) -> ()  [unwired: 1 out]
      }
      frame True {
        # "Here is where you would annotate,\npossibly process, and display the image"
        # "Update Mbps LED"
        n89 = call "IMAQ Clear Overlay"("Image"=w205) -> ("error out"=w206:errorcluster, "Image Out"=w204:T5)  [unwired: 2 in, 7 out]
        n90 = Unbundle By Name(w206) -> ("status"=w207:bool)
        n91 = property on="Image Message" class="Str"("Visible"=w207) -> ()  [unwired: 2 in, 2 out]
      }
    }
    "Camera Image" <- w194
    n92 = call <vilib>:"WPI_DashboardFormatPerf.vi"("Right Camera Perf"=w187, "Performance"=w188, "String in"=w186) -> ()  [unwired: 9 in]
  }
  n93 = call "Handle Camera Configuration.vi"("CameraNameRef"=w35, "Display Name"=w28, "ClusterRef"=w36) -> ()  [unwired: 9 in]
  n94 = while {
    tunnel: w38 -> [w222]
    tunnel: w37 -> [_]
    tunnel: [w217] -> _
    tunnel: w29 -> [w213]
    tunnel: w28 -> [w210]
    i -> [w217]
    stop <- FALSE stop-if-true
    n95 = local read "NT Connection"() -> (w214:bool)
    n96 = local read "Rec Mode"() -> (w221:enum32{"Stop", "Record", "Playback"})
    n97 = Bundle("Camera Name Right"="Camera Name Right", w210, "Saved DB Images Info"=w213) -> (w212:T21)  [unwired: 1 in]
    n98 = call <vilib>:"WPI_CameraRead MJPG for Dashboard_2.vi"("Camera Settings"="Camera Settings Right", "Rec Mode"=w221, "NT Connection"=w214, "Capture Info"=w212, "Image in"=w222) -> ("perf info"=w208:cluster{"Bandwidth (Mbps)":dbl, "fps":dbl}, "Active"=w216:bool, "Image\\ out"=w219:T5)  [unwired: 4 in]
    n99 = case shown="True" w216 {
      tunnel: w219 -> [w224 w227]
      tunnel: [w224 w227] -> w215
      tunnel: [_ w226] -> w209
      tunnel: w208 -> [_ w226]
      frame False {
        n100 = Wait Until Next ms Multiple(millisecond multiple=u32 500) -> ()  [unwired: 1 out]
        n101 = property on="Camera Image Right" class="ImageControl"("ROI"=T19 {"Global Rectangle"=[], "Contours"=[]}) -> ()  [unwired: 2 in, 2 out]
      }
      frame True {
      }
    }
    "Camera Image Right" <- w215
    "Right Camera Perf" <- w209
  }
  n102 = register-events(refnum<vi> refnum, w51) -> (reference out=w89:refnum<event-registration>, error out=w88:errorcluster)  [unwired: 2 in]
  n103 = call "Initialize Camera and CheckList.vi"("ListBox in"=w73) -> ()  [unwired: 11 in]
  n104 = call "Adjust Dashboard Window.vi"("Sizing Refnums"=w74, "Size Constraints"=w76, "VI"=w84, "WIn Mode"=w60) -> ()  [unwired: 8 in]
  n105 = while {
    tunnel: w81 -> [w239]
    tunnel: w61 -> [w237]
    tunnel: [w235] -> _
    tunnel: u32 1000 ("milliseconds to wait") -> [w234]
    tunnel: w51 -> [w228]
    i -> [w235]
    stop <- FALSE stop-if-true
    n106 = local read "Rec Mode"() -> (w230:enum32{"Stop", "Record", "Playback"})
    n107 = Wait on Notification(notifier=w237, timeout in ms (-1)=w234) -> (notification=w236:string, timed out?=w232:bool)  [unwired: 2 in, 2 out]
    n108 = Equal?(x=w230, y=u16 2 ("Rec Mode")) -> (x = y?=w231:bool)
    n109 = Compound Arithmetic op=OR(invert w232, w231) -> (w233:bool)
    n110 = case shown="True" w233 {
      tunnel: w239 -> [_ w242]
      tunnel: w236 -> [_ w241]
      tunnel: w228 -> [_ w240]
      frame False {
      }
      frame True {
        n111 = call <vilib>:"Bind Controls to SmartDashboard.vi"("RPC ref"=w240, "Bound Control Refs"=w242, "Server IP Address"=w241) -> ()  [unwired: 9 in]
      }
    }
  }
  n112 = vi-ref "Playback Controls.vi"() -> (w90:refnum<vi>)
  n113 = property class="VI"() -> ("Panel"=w92:refnum<vi>)  [unwired: 2 in, 2 out]
  n114 = property class="Pnl"(reference=w92) -> ("Panes[]"=w93:refnum<vi>[])  [unwired: 1 in, 2 out]
  n115 = Index Array(array=w93) -> (element=w91:refnum<vi>)  [unwired: 1 in]
  n116 = control-ref of="Test Tree"() -> (w94:refnum<vi>)
  n117 = while {
    tunnel: [w252] -> _
    tunnel: w94 -> [w251]
    tunnel: w90 -> [w250]
    tunnel: w89 -> [w249]
    tunnel: w88 -> [_]
    tunnel: w84 -> [w248]
    tunnel: w51 -> [w247]
    tunnel: w49 -> [w246]
    shift-right: [w245] -> _
    shift-left: _ -> [w244]
    tunnel: w43 -> [w243]
    i -> [w252]
    stop <- FALSE stop-if-true
    n118 = event shown="[0] Timeout" {
      selector: w249 -> [_ _ _ _ _ _ _ _ _ _ _ _ _ _ _ _ _ _ _ _ _]
      dyn-events: [_ _ _ _ _ _ _ _ _ _ _ _ _ _ _ _ w512 _ _ _ _] -> _
      timeout: u32 60 ("milliseconds to wait") -> [_ _ _ _ _ _ _ _ _ _ _ _ _ _ _ _ _ _ _ _ _]
      tunnel: w251 -> [w264 _ _ _ _ _ _ _ _ _ _ _ _ _ _ _ _ _ _ _ _]
      tunnel: "Test Tree" -> [_ _ _ _ _ _ _ _ _ _ _ w479 w487 w489 w493 w501 _ _ _ _ _]
      tunnel: w250 -> [_ _ _ _ _ _ _ _ _ _ _ _ _ _ _ _ w514 _ w532 _ _]
      tunnel: w248 -> [_ _ _ _ _ _ _ _ _ _ _ _ _ _ _ _ w510 _ _ _ _]
      tunnel: w247 -> [_ _ _ _ _ _ _ _ _ _ _ _ _ _ _ _ w508 _ _ _ _]
      tunnel: w246 -> [w259 _ _ _ _ _ w430 _ _ _ _ _ _ _ _ _ _ _ _ _ _]
      tunnel: [w258 w307 w409 w414 w423 w427 w428 w437 w447 w454 w466 w478 w485 w488 w492 w500 w507 w527 w529 w533 w546] -> w245
      tunnel: w244 -> [w258 w307 w409 w414 w423 w427 w428 _ _ w454 w466 w478 w485 w488 w492 w500 w507 w527 w529 w533 w546]
      tunnel: w243 -> [w256 _ _ _ _ _ _ _ _ _ _ _ _ _ _ _ _ _ _ _ _]
      event Timeout {
        n119 = event-data() -> ()  [unwired: 1 in, 1 out]
        n120 = local read "Mode"() -> (w261:T4)
        n121 = case shown="\"Test\"" "Dashboard Tab" {
          tunnel: w264 -> [_ _ w280 _ _]
          tunnel: "TestMode/Automatic/" ("Name Pattern") -> [_ _ w279 _ _]
          tunnel: T22 [{"Operation"=enum."Clear", "Color Box"=14013909}, {"Operation"=enum."Clear", "Color Box"=14013909}, {"Operation"=enum."Clear", "Color Box"=14013909}, {"Operation"=enum."Clear", "Color Box"=14013909}, {"Operation"=enum."Update", "Color Box"=14013909}, {"Operation"=enum."Update", "Color Box"=16777215}, {"Operation"=enum."Clear", "Color Box"=14013909}, {"Operation"=enum."Clear", "Color Box"=14013909}, {"Operation"=enum."Clear", "Color Box"=14013909}] -> [_ _ w272 _ w300]
          tunnel: w261 -> [_ _ w271 _ w299]
          tunnel: u32[] [15790320, 15790320, 15790320, 15790320, 16777215, 16777215, 15790320, 15790320, 15790320] -> [_ _ _ _ w305]
          tunnel: w259 -> [_ _ _ _ w293]
          tunnel: w256 -> [_ w266 _ _ _]
          frame "Custom", Default {
          }
          frame "Basic" {
            n122 = call <vilib>:"WPI_DashboardUpdateNames.vi"("Controls on Tab"=w266) -> ()  [unwired: 11 in]
          }
          frame "Test" {
            w278 = -2 ("Active Item:Row Number")
            n123 = Index Array(array=w272, index=w271) -> (element=w273:T25)
            n124 = Unbundle(w273) -> ("Operation"=w274:enum16{"Update", "Clear"}, "Color Box"=w275:u32)
            n125 = call <vilib>:"NT Read String.vi"("Name"="TestMode/TestName") -> ("String"=w269:string)  [unwired: 9 in, 1 out]
            n126 = call <vilib>:"NT Read and Format Entries as Tree.vi"("Operation"=w274, "Name Pattern"=w279, "Tree Refnum"=w280) -> ()  [unwired: 7 in, 2 out]
            n127 = case shown="\"\"" w269 {
              tunnel: "TestMode/TestProgress" ("Name") -> [w282 _]
              tunnel: "TestMode/TestProgressText" ("Name") -> [w281 _]
              frame Default {
                n128 = call <vilib>:"NT Read Number.vi"("Name"=w282) -> ("Numeric"=w283:dbl)  [unwired: 9 in, 1 out]
                n129 = call <vilib>:"NT Read String.vi"("Name"=w281) -> ("String"=w284:string)  [unwired: 9 in, 1 out]
                n130 = Bundle("Numeric"=w283, "String"=w284) -> (→"Progress":cluster{"Numeric":dbl, "String":string})  [unwired: 1 in]
              }
              frame "" {
                n131 = property on="Progress" class="Clust (strict)"("Visible"=FALSE) -> ()  [unwired: 2 in, 2 out]
                n132 = local write "Test Name"(u16 0) -> ()
              }
            }
            n133 = property on="Test Tree" class="Tree (strict)"("Active Item Row Number"=w278, "ActiveColNum"=w278, "CellBG"=w275, "Active Item Row Number"=-1 ("Active Item:Row Number"), "CellBG"=u32 5789784 ("Color Box")) -> ()  [unwired: 2 in, 2 out]
          }
          frame "Variables" {
            w290 = string[] ["CameraPublisher", "Usage", "DB"]  # Items to initially close
            n134 = First Call?() -> (First Call?: T/F=w291:bool)
            n135 = control-ref of="Tree"() -> (w292:refnum<vi>)
            n136 = Select(t=w290, s=w291, f=string[] []) -> (s? t:f=w288:string[])
            n137 = call <vilib>:"NT Read and Format Entries as Tree.vi"("Tags to  Close"=w288, "Tree Refnum"=w292) -> ()  [unwired: 8 in, 2 out]
          }
          frame "Commands" {
            w301 = u32 5789784 ("Color Box")
            w302 = T26 {"Row"=-1, "Column"=-2} ("Active Cell:Active Cell")
            w304 = T26 {"Row"=-2, "Column"=-2} ("Active Cell:Active Cell")
            n138 = Index Array(array=w305, index=w299) -> (element=w303:u32)
            n139 = Index Array(array=w300, index=w299) -> (element=w298:T25)
            n140 = Unbundle(w298) -> ("Operation"=w297:enum16{"Update", "Clear"})  [unwired: 1 out]
            n141 = local read "Command Selection"() -> (w296:i32)
            n142 = property on="Command Selection" class="MCListbox (strict)"("ActiveCell"=w304, "CellBG"=w303, "ActiveCell"=w302, "CellBG"=w301) -> ()  [unwired: 2 in, 2 out]
            n143 = call <vilib>:"WPI_DashboardUpdate RPC Info.vi"("Operation"=w297) -> ("update"=w295:bool, "commands"=w294:string[][])  [unwired: 9 in]
            n144 = property on="Command Selection" class="MCListbox (strict)"("ItemNames"=w294) -> ()  [unwired: 2 in, 2 out]
            n145 = property on="Command Params" class="Tbl (strict)"("Active Cell"=w304, "Cell BG Color"=w303, "Active Cell"=w302, "Cell BG Color"=w301) -> ()  [unwired: 2 in, 2 out]
            n146 = call <vilib>:"WPI_DashboardUpdate Command Params.vi"("Update"=w295, "NewVal"=w296, "Commands"=w294, "Param Tbl"=w293) -> ()  [unwired: 7 in, 1 out]
          }
        }
        n147 = call <vilib>:"Connextion Info.vi"() -> ("Connected"=→"NT Connection":bool)  [unwired: 10 in, 1 out]
      }
      event "Test Tree": Value Change {
        # "Show appropriate\ncontrols"
        n148 = event-data() -> ("CtlRef"=w310:refnum<vi>, "NewVal"=w308:string)  [unwired: 1 in]
        n149 = call <vilib>:"WPI_UtilitiesGetTreeIOName.vi"("NewVal"=w308, "TreeControl in"=w310) -> ("I/O Name"=w311:string)  [unwired: 9 in]
        n150 = case shown="\"Camera\"" w311 {
          selector: w311 -> [_ w318 _ w340 w349 _]
          tunnel: w308 -> [_ _ w337 w339 _ w356]
          tunnel: cluster{string[]}[] [{["640x480", "320x240", "160x120"]}, {["Auto", "Fixed indoor", "Fixed outdoor 1", "Fixed outdoor 2", "Fixed fluorescent 1", "Fixed fluorescent 2", "Hold current"]}, {["Auto", "Flicker-free 50 Hz", "Flicker-free 60 Hz", "Hold current"]}, {["None", "Prioritize frame rate", "Prioritize image quality"]}, {["Monochrome", "Color"]}] -> [_ _ _ _ _ w355]
          frame Default {
            w313 = FALSE ("Visible")
            w312 = FALSE ("Visible")
            n151 = property on="Motor" class="Clust (strict)"("Visible"=w312) -> ()  [unwired: 2 in, 2 out]
            n152 = property on="Test Ring" class="Ring (strict)"("Visible"=w312) -> ()  [unwired: 2 in, 2 out]
            n153 = property on="Rev/Fwd" class="Clust (strict)"("Visible"=w313) -> ()  [unwired: 2 in, 2 out]
            n154 = property on="On/Off" class="Bool (strict)"("Visible"=w313) -> ()  [unwired: 2 in, 2 out]
            n155 = property on="Test Slider" class="Slide (strict)"("Visible"=w313) -> ()  [unwired: 2 in, 2 out]
          }
          frame "Analog Out", "Motor", "PWM" {
            w319 = FALSE ("Visible")
            n156 = case shown="\"Analog Out\"" w318 {
              tunnel: [1.0 ("Value") -1.0 ("Value") 0.0 ("Value")] -> w317
              tunnel: [255.0 ("Value") 1.0 ("Value") 5.0 ("Value")] -> w316
              tunnel: [128.0 ("Value") 0.0 ("Value") 0.0 ("Value")] -> w315
              tunnel: [64.0 ("Value") 0.5 ("Value") 1.0 ("Value")] -> w314
              frame "PWM" {
              }
              frame "Motor", Default {
              }
              frame "Analog Out" {
              }
            }
            n157 = property on="Motor" class="Clust (strict)"("Visible"=TRUE) -> ()  [unwired: 2 in, 2 out]
            n158 = property on="Value" class="Slide (strict)"("Value"=w315, "Scale.Minimum"=w317, "Scale.Maximum"=w316, "Scale.Increment"=w314) -> ()  [unwired: 2 in, 2 out]
            n159 = property on="On/Off" class="Bool (strict)"("Visible"=w319) -> ()  [unwired: 2 in, 2 out]
            n160 = property on="Test Slider" class="Slide (strict)"("Visible"=w319) -> ()  [unwired: 2 in, 2 out]
            n161 = property on="Test Ring" class="Ring (strict)"("Visible"=w319) -> ()  [unwired: 2 in, 2 out]
            n162 = property on="Rev/Fwd" class="Clust (strict)"("Visible"=w319) -> ()  [unwired: 2 in, 2 out]
          }
          frame "Servo" {
            w335 = FALSE ("Visible")
            n163 = call <vilib>:"NT Read Number.vi"("Name"=w337) -> ("Numeric"=w336:dbl)  [unwired: 9 in, 1 out]
            n164 = property on="Test Slider" class="Slide (strict)"("Visible"=TRUE, "Scale.Maximum"=170.0 ("Scale.Range:Maximum")) -> ()  [unwired: 2 in, 2 out]
            n165 = local write "Test Slider"(w336) -> ()
            n166 = property on="Motor" class="Clust (strict)"("Visible"=w335) -> ()  [unwired: 2 in, 2 out]
            n167 = property on="Rev/Fwd" class="Clust (strict)"("Visible"=w335) -> ()  [unwired: 2 in, 2 out]
            n168 = property on="On/Off" class="Bool (strict)"("Visible"=w335) -> ()  [unwired: 2 in, 2 out]
            n169 = property on="Test Ring" class="Ring (strict)"("Visible"=w335) -> ()  [unwired: 2 in, 2 out]
          }
          frame "Relay", "Solenoid" {
            w338 = FALSE ("Visible")
            n170 = property on="Motor" class="Clust (strict)"("Visible"=w338) -> ()  [unwired: 2 in, 2 out]
            n171 = property on="Test Slider" class="Slide (strict)"("Visible"=w338) -> ()  [unwired: 2 in, 2 out]
            n172 = Search and Replace String(input string=w339, search string="/Value  **", replace string="/Direction") -> (result string=w345:string)  [unwired: 5 in, 3 out]
            n173 = property on="Test Ring" class="Ring (strict)"("Visible"=w338) -> ()  [unwired: 2 in, 2 out]
            n174 = call <vilib>:"NT Read String.vi"("Name"=w345) -> ("String"=w343:string)  [unwired: 9 in, 1 out]
            n175 = Equal?(x="Both directions", y=w343) -> (x = y?=w341:bool)
            n176 = Not(x=w341) -> (.not. x?=w342:bool)
            n177 = property on="Rev/Fwd" class="Clust (strict)"("Visible"=w341) -> ()  [unwired: 2 in, 2 out]
            n178 = property on="On/Off" class="Bool (strict)"("Visible"=w342, "Caption.Text"=w340) -> ()  [unwired: 2 in, 2 out]
          }
          frame "Compressor", "Digital Out" {
            w348 = FALSE ("Visible")
            # "Get direction and finish"
            n179 = property on="Motor" class="Clust (strict)"("Visible"=w348) -> ()  [unwired: 2 in, 2 out]
            n180 = property on="Test Slider" class="Slide (strict)"("Visible"=w348) -> ()  [unwired: 2 in, 2 out]
            n181 = property on="Test Ring" class="Ring (strict)"("Visible"=w348) -> ()  [unwired: 2 in, 2 out]
            n182 = property on="On/Off" class="Bool (strict)"("Visible"=TRUE, "Caption.Text"=w349) -> ()  [unwired: 2 in, 2 out]
            n183 = property on="Rev/Fwd" class="Clust (strict)"("Visible"=FALSE) -> ()  [unwired: 2 in, 2 out]
          }
          frame "Camera" {
            n184 = call <vilib>:"Get Last Path Segment.vi"("String in"=w356) -> ("String out"=w357:string)  [unwired: 10 in]
            n185 = property on="On/Off" class="Bool (strict)"("Visible"=FALSE) -> ()  [unwired: 2 in, 2 out]
            n186 = property on="Motor" class="Clust (strict)"("Visible"=FALSE) -> ()  [unwired: 2 in, 2 out]
            n187 = property on="Rev/Fwd" class="Clust (strict)"("Visible"=FALSE) -> ()  [unwired: 2 in, 2 out]
            n188 = case shown="\"White Balance  **\"" w357 {
              tunnel: w356 -> [w363 w372 w381 w390 w399 _ w405]
              tunnel: w355 -> [w361 w369 w378 w387 w396 _ _]
              frame "Size  **" {
                n189 = Index Array(array=w361) -> (element=w360:cluster{string[]})  [unwired: 1 in]
                n190 = call <vilib>:"NT Read String.vi"("Name"=w363) -> ("String"=w362:string)  [unwired: 9 in, 1 out]
                n191 = Unbundle(w360) -> (w358:string[])
                n192 = Match First String(2:w358, 3:w362) -> (0:w359:i32)  [unwired: 1 out]
                n193 = property on="Test Ring" class="Ring (strict)"("Value"=w359, "Strings []"=w358) -> ()  [unwired: 2 in, 2 out]
                n194 = property on="Test Ring" class="Ring (strict)"("Visible"=TRUE) -> ()  [unwired: 2 in, 2 out]
                n195 = property on="Test Slider" class="Slide (strict)"("Visible"=FALSE) -> ()  [unwired: 2 in, 2 out]
              }
              frame "White Balance  **" {
                n196 = Index Array(array=w369, index=1) -> (element=w370:cluster{string[]})
                n197 = call <vilib>:"NT Read String.vi"("Name"=w372) -> ("String"=w371:string)  [unwired: 9 in, 1 out]
                n198 = Unbundle(w370) -> (w367:string[])
                n199 = Match First String(2:w367, 3:w371) -> (0:w366:i32)  [unwired: 1 out]
                n200 = property on="Test Ring" class="Ring (strict)"("Value"=w366, "Strings []"=w367) -> ()  [unwired: 2 in, 2 out]
                n201 = property on="Test Ring" class="Ring (strict)"("Visible"=TRUE) -> ()  [unwired: 2 in, 2 out]
                n202 = property on="Test Slider" class="Slide (strict)"("Visible"=FALSE) -> ()  [unwired: 2 in, 2 out]
              }
              frame "Exposure  **" {
                n203 = Index Array(array=w378, index=2) -> (element=w379:cluster{string[]})
                n204 = call <vilib>:"NT Read String.vi"("Name"=w381) -> ("String"=w380:string)  [unwired: 9 in, 1 out]
                n205 = Unbundle(w379) -> (w375:string[])
                n206 = Match First String(2:w375, 3:w380) -> (0:w376:i32)  [unwired: 1 out]
                n207 = property on="Test Ring" class="Ring (strict)"("Value"=w376, "Strings []"=w375) -> ()  [unwired: 2 in, 2 out]
                n208 = property on="Test Ring" class="Ring (strict)"("Visible"=TRUE) -> ()  [unwired: 2 in, 2 out]
                n209 = property on="Test Slider" class="Slide (strict)"("Visible"=FALSE) -> ()  [unwired: 2 in, 2 out]
              }
              frame "Exposure Priority  **" {
                n210 = Index Array(array=w387, index=3) -> (element=w388:cluster{string[]})
                n211 = call <vilib>:"NT Read String.vi"("Name"=w390) -> ("String"=w389:string)  [unwired: 9 in, 1 out]
                n212 = Unbundle(w388) -> (w384:string[])
                n213 = Match First String(2:w384, 3:w389) -> (0:w385:i32)  [unwired: 1 out]
                n214 = property on="Test Ring" class="Ring (strict)"("Value"=w385, "Strings []"=w384) -> ()  [unwired: 2 in, 2 out]
                n215 = property on="Test Ring" class="Ring (strict)"("Visible"=TRUE) -> ()  [unwired: 2 in, 2 out]
                n216 = property on="Test Slider" class="Slide (strict)"("Visible"=FALSE) -> ()  [unwired: 2 in, 2 out]
              }
              frame "Color Enable  **" {
                n217 = Index Array(array=w396, index=4) -> (element=w397:cluster{string[]})
                n218 = call <vilib>:"NT Read String.vi"("Name"=w399) -> ("String"=w398:string)  [unwired: 9 in, 1 out]
                n219 = Unbundle(w397) -> (w393:string[])
                n220 = Match First String(2:w393, 3:w398) -> (0:w394:i32)  [unwired: 1 out]
                n221 = property on="Test Ring" class="Ring (strict)"("Value"=w394, "Strings []"=w393) -> ()  [unwired: 2 in, 2 out]
                n222 = property on="Test Ring" class="Ring (strict)"("Visible"=TRUE) -> ()  [unwired: 2 in, 2 out]
                n223 = property on="Test Slider" class="Slide (strict)"("Visible"=FALSE) -> ()  [unwired: 2 in, 2 out]
              }
              frame Default {
                n224 = property on="Test Ring" class="Ring (strict)"("Visible"=FALSE) -> ()  [unwired: 2 in, 2 out]
                n225 = property on="Test Slider" class="Slide (strict)"("Visible"=FALSE) -> ()  [unwired: 2 in, 2 out]
              }
              frame "Brightness  **", "Color Level  **", "Compression  **", "FPS  **", "Sharpness  **" {
                n226 = call <vilib>:"NT Read Number.vi"("Name"=w405) -> ("Numeric"=w404:dbl)  [unwired: 9 in, 1 out]
                n227 = local write "Test Slider"(w404) -> ()
                n228 = property on="Test Slider" class="Slide (strict)"("Visible"=TRUE, "Scale.Maximum"=100.0 ("Scale.Range:Maximum")) -> ()  [unwired: 2 in, 2 out]
                n229 = property on="Test Ring" class="Ring (strict)"("Visible"=FALSE) -> ()  [unwired: 2 in, 2 out]
              }
            }
          }
        }
        n230 = property on="Progress" class="Clust (strict)"("Visible"=FALSE) -> ()  [unwired: 2 in, 2 out]
      }
      event "Test Name": Mouse Enter {
        # "Populate the ring with the list of tests"
        n231 = event-data() -> ()  [unwired: 1 in, 1 out]
        n232 = call <vilib>:"NT Read String Array.vi"("Name"="TestMode/TestList") -> ("String Array"=w413:string[])  [unwired: 9 in, 1 out]
        n233 = Build Array (concatenate)("Select the test to run...", w413) -> (w412:string[])
        n234 = property on="Test Name" class="Ring (strict)"("Strings []"=w412) -> ()  [unwired: 2 in, 2 out]
      }
      event "Test Name": Value Change {
        w415 = FALSE ("Visible")
        # "Tell the robot the test name to run"
        n235 = event-data() -> ("NewVal"=w419:u16)  [unwired: 1 in]
        n236 = property on="Test Name" class="Ring (strict)"() -> ("Strings []"=w420:string[])  [unwired: 2 in, 2 out]
        n237 = local write "Progress"(T6 {"Test Progress"=0, "Test Progress Text"=""} ("Progress")) -> ()
        n238 = Index Array(array=w420, index=w419) -> (element=w418:string)
        n239 = call <vilib>:"NT Write String.vi"("String"=w418, "Name"="TestMode/TestName") -> ()  [unwired: 9 in, 1 out]
        n240 = property on="Progress" class="Clust (strict)"("Visible"=TRUE) -> ()  [unwired: 2 in, 2 out]
        n241 = property on="Motor" class="Clust (strict)"("Visible"=w415) -> ()  [unwired: 2 in, 2 out]
        n242 = property on="Test Slider" class="Slide (strict)"("Visible"=w415) -> ()  [unwired: 2 in, 2 out]
        n243 = property on="On/Off" class="Bool (strict)"("Visible"=w415) -> ()  [unwired: 2 in, 2 out]
        n244 = property on="Rev/Fwd" class="Clust (strict)"("Visible"=w415) -> ()  [unwired: 2 in, 2 out]
        n245 = property on="Test Ring" class="Ring (strict)"("Visible"=w415) -> ()  [unwired: 2 in, 2 out]
      }
      event "Select Auto": Mouse Enter {
        # "Populate the combo box with the list of autonomous options"
        n246 = event-data() -> ()  [unwired: 1 in, 1 out]
        n247 = call <vilib>:"NT Read String Array.vi"("Name"="Auto List") -> ("String Array"=w422:string[])  [unwired: 9 in, 1 out]
        n248 = property on="Select Auto" class="CmbBox"("Strings[]"=w422) -> ()  [unwired: 2 in, 2 out]
      }
      event "Select Auto": Value Change {
        # "User modified the Auto Selection. Write to NT variable so robot knows."
        n249 = event-data() -> ("NewVal"=w425:string)  [unwired: 1 in]
        n250 = call <vilib>:"NT Write String.vi"("String"=w425, "Name"="Auto Selector") -> ()  [unwired: 9 in, 1 out]
      }
      event "Command Selection": Value Change {
        # "Get the params and show in table"
        n251 = event-data() -> ("NewVal"=w431:i32)  [unwired: 1 in]
        n252 = property on="Command Selection" class="MCListbox (strict)"() -> ("ItemNames"=w429:string[][])  [unwired: 2 in, 2 out]
        n253 = call <vilib>:"WPI_DashboardUpdate Command Params.vi"("NewVal"=w431, "Commands"=w429, "Param Tbl"=w430) -> ()  [unwired: 8 in, 1 out]
      }
      event "Execute Command": Value Change {
        # "Started one, Unique ID holds\nresponse"
        n254 = event-data() -> ()  [unwired: 1 in, 1 out]
        n255 = property on="Command Selection" class="MCListbox (strict)"() -> ("ItemNames"=w442:string[][])  [unwired: 2 in, 2 out]
        n256 = Index Array(array=w442, index (row)="Command Selection", index (col)=0) -> (element=w440:string)
        n257 = call <vilib>:"Invoke Commands.vi"("Command Params"="Command Params", "Function Name"=w440) -> ("Params"=w436:u8, "Started"=w435:bool)  [unwired: 7 in, 1 out]
        n258 = Array Subset(array="Command Params", length (row)=w436) -> (w437:string[][])  [unwired: 3 in]
        n259 = Select(t="Executing" ("Cmd Status"), s=w435, f="" ("Cmd Status")) -> (s? t:f=→"Cmd Status":string)
      }
      event "Command Selection": Double Click {
        n260 = event-data() -> ("Row"=w450:i32)  [unwired: 1 in]
        n261 = property on="Command Selection" class="MCListbox (strict)"() -> ("ItemNames"=w453:string[][])  [unwired: 2 in, 2 out]
        n262 = local read "Command Params"() -> (w449:string[][])
        n263 = Index Array(array=w453, index (row)=w450, index (col)=0) -> (element=w451:string)
        n264 = call <vilib>:"Invoke Commands.vi"("Command Params"=w449, "Function Name"=w451) -> ("Params"=w448:u8, "Started"=w443:bool)  [unwired: 7 in, 1 out]
        n265 = Array Subset(array=w449, length (row)=w448) -> (w447:string[][])  [unwired: 3 in]
        n266 = Select(t="Executing" ("Cmd Status"), s=w443, f="" ("Cmd Status")) -> (s? t:f=w444:string)
        n267 = local write "Cmd Status"(w444) -> ()
      }
      event "CheckList": Double Click {
        # "Shift clears all"
        # "Update symbols on the listbox"
        n268 = event-data() -> ("PlatMods.Shift"=w455:bool, "Row"=w457:i32)  [unwired: 1 in]
        n269 = case shown="True" w455 {
          tunnel: w457 -> [w461 _]
          tunnel: 1 -> [w460 _]
          frame False {
            n270 = property on="CheckList" class="LstBox (strict)"() -> ("Item Symbols"=w459:i32[])  [unwired: 2 in, 2 out]
            n271 = Replace Array Subset(array=w459, new element=w460, index=w461) -> (w458:i32[])
            n272 = property on="CheckList" class="LstBox (strict)"("Item Symbols"=w458) -> ()  [unwired: 2 in, 2 out]
          }
          frame True {
            w462 = 0 ("Top Row")
            n273 = property on="CheckList" class="LstBox (strict)"() -> ("Number of Rows"=w464:u32)  [unwired: 2 in, 2 out]
            n274 = Initialize Array(0, w464) -> (w463:i32[])
            n275 = property on="CheckList" class="LstBox (strict)"("Top Row"=w462, "Value"=w462, "Item Symbols"=w463) -> ()  [unwired: 2 in, 2 out]
          }
        }
      }
      event "CheckList": Key Down {
        # "Update symbols on the listbox\nLeft and right keys check and uncheck"
        n276 = event-data() -> ("VKey"=w468:T23)  [unwired: 1 in]
        n277 = case shown="\"Left\", \"Right\"" w468 {
          selector: w468 -> [w473 _]
          tunnel: eventvkey."Left" ("VKey") -> [w471 _]
          frame "Left", "Right" {
            n278 = Equal?(x=w471, y=w473) -> (x = y?=w472:bool)
            n279 = Select(t=0, s=w472, f=1) -> (s? t:f=w474:i32)
            n280 = property on="CheckList" class="LstBox (strict)"() -> ("Item Symbols"=w477:i32[])  [unwired: 2 in, 2 out]
            n281 = Replace Array Subset(array=w477, new element=w474, index="CheckList") -> (w476:i32[])
            n282 = property on="CheckList" class="LstBox (strict)"("Item Symbols"=w476) -> ()  [unwired: 2 in, 2 out]
          }
          frame Default {
          }
        }
      }
      event "Motor.Enable": Value Change {
        # "When the test mode otor enable helper is set, update that\ntree row item's value"
        n283 = event-data() -> ("NewVal"=w483:bool)  [unwired: 1 in]
        n284 = Unbundle("Motor") -> ("Value"=w482:dbl)  [unwired: 1 out]
        n285 = Select(t=w482, s=w483, f=0.0) -> (s? t:f=w480:dbl)
        n286 = call <vilib>:"NT Write Number.vi"("Numeric"=w480, "Name"=w479) -> ()  [unwired: 9 in, 1 out]
      }
      event "Test Slider": Value Change {
        # "When the test mode slider helper is set, update that\ntree row item's value"
        n287 = event-data() -> ("NewVal"=w486:dbl)  [unwired: 1 in]
        n288 = call <vilib>:"NT Write Number.vi"("Numeric"=w486, "Name"=w487) -> ()  [unwired: 9 in, 1 out]
      }
      event "On/Off": Value Change {
        # "When the test mode on/off helper value is set, update that\ntree row item's value"
        n289 = event-data() -> ("NewVal"=w491:bool)  [unwired: 1 in]
        n290 = Boolean To (0,1)(Boolean=w491) -> (0, 1=w490:i16)
        n291 = call <vilib>:"NT Write Number.vi"("Numeric"=w490, "Name"=w489) -> ()  [unwired: 9 in, 1 out]
      }
      event "Rev/Fwd": Value Change {
        # "When the test mode helper value for relays is set, update that\ntree row item's value"
        n292 = event-data() -> ("NewVal.Forward"=w499:bool, "NewVal.Reverse"=w498:bool)  [unwired: 1 in]
        n293 = Boolean To (0,1)(Boolean=w499) -> (0, 1=w495:i16)
        n294 = Boolean To (0,1)(Boolean=w498) -> (0, 1=w497:i16)
        n295 = Negate(x=w497) -> (-x=w496:i16)
        n296 = Add(x=w495, y=w496) -> (x+y=w494:i16)
        n297 = call <vilib>:"NT Write Number.vi"("Numeric"=w494, "Name"=w493) -> ()  [unwired: 9 in, 1 out]
      }
      event "Test Ring": Value Change {
        # "When a test mode helper value is selected from the ring,\nset the tree item's variable to the string value"
        n298 = event-data() -> ("NewVal"=w503:u16)  [unwired: 1 in]
        n299 = property on="Test Ring" class="Ring (strict)"() -> ("Strings []"=w504:string[])  [unwired: 2 in, 2 out]
        n300 = Index Array(array=w504, index=w503) -> (element=w502:string)
        n301 = call <vilib>:"NT Write String.vi"("String"=w502, "Name"=w501) -> ()  [unwired: 9 in, 1 out]
      }
      event "Rec Mode": Value Change {
        # "Update globals for recording mode and path to read log from.\nClear when logging and let NetworkTables set path for vision to\nuse."
        n302 = event-data() -> ("NewVal"=w515:enum32{"Stop", "Record", "Playback"})  [unwired: 1 in]
        n303 = global write "WPI_DashboardLogging Global.vi" "Logging Filename"(path "") -> ()
        n304 = global write "WPI_DashboardLogging Global.vi" "Recording"(w515) -> ()
        n305 = case shown="\"Playback\"" w515 {
          tunnel: w514 -> [_ w517 w526]
          tunnel: [_ _ w525] -> w512
          tunnel: [_ _ w524] -> _
          tunnel: w510 -> [_ _ w522]
          tunnel: cluster{i32, i32} {-250, 170} -> [_ _ w521]
          tunnel: [_ _ T24 {"Image Size"=TRUE, "Image Type"=TRUE, "Pixel Value"=TRUE, "ROI Information"=TRUE, "Zoom Factor"=FALSE} ("Image Information Shown:All Elements")] -> w505
          tunnel: [_ _ TRUE ("Zoom Factor")] -> w506
          tunnel: w508 -> [_ _ w518]
          frame Default {
          }
          frame "Stop", "Record" {
            # "Place Window too"
            n306 = invoke class="VI" method="FP.Close"(reference=w517) -> (reference out=w516:refnum<vi>)  [unwired: 2 in, 2 out]
            n307 = invoke class="VI" method="Abort VI"(reference=w516) -> ()  [unwired: 2 in, 3 out]
          }
          frame "Playback" {
            n308 = call "Open Playback Panel.vi"("Offset"=w521, "DB VI Ref"=w522, "Playback in"=w526) -> ("Playback out"=w523:refnum<vi>)  [unwired: 8 in]
            n309 = register-events(w523, w518) -> (reference out=w525:refnum<event-registration>, error out=w524:errorcluster)  [unwired: 2 in]
          }
        }
        n310 = property on="Camera Image Right" class="ImageControl"("Image Information Shown"=w505, "Image Information Visible"=w506) -> ()  [unwired: 2 in, 2 out]
        n311 = property on="Camera Image" class="ImageControl"("Image Information Shown"=w505, "Image Information Visible"=w506) -> ()  [unwired: 2 in, 2 out]
        n312 = call <vilib>:"WPI_DashboardNT Log FieldName Cache.vi"("Operation"=enum16{"Lookup/Add", "Index", "Clear"}."Clear") -> ()  [unwired: 8 in, 3 out]
      }
      event Panel Close {
        w528 = enum32{"Stop", "Record", "Playback"}."Stop" ("Rec Mode")
        # "Playback window has been closed, abort"
        n313 = event-data() -> ()  [unwired: 1 in, 4 out]
        n314 = local write "Rec Mode"(w528) -> ()
        n315 = global write "WPI_DashboardLogging Global.vi" "Recording"(w528) -> ()
      }
      event Panel Close {
        # "Abort playback window and ourself"
        n316 = event-data() -> ()  [unwired: 1 in, 4 out]
        n317 = invoke class="VI" method="FP.Close"(reference=w532) -> (reference out=w531:refnum<vi>)  [unwired: 2 in, 2 out]
        n318 = invoke class="VI" method="Abort VI"(reference=w531) -> (error out=w530:errorcluster)  [unwired: 2 in, 2 out]
        n319 = invoke class="VI" method="Abort VI"(error in=w530) -> ()  [unwired: 2 in, 3 out]
      }
      event User Event {
        n320 = event-data() -> ("IDs"=w539:cluster{"RPC field ID":u16, "Unique ID":u16}, "String"=w538:string)  [unwired: 1 in]
        n321 = Bundle("IDs"=w539, "String"=w538) -> (w537:T10)  [unwired: 1 in]
        n322 = call <vilib>:"Retrieve RPC Response.vi"("RPC Response"=w537) -> ("Output"=w535:string[][])  [unwired: 10 in]
        n323 = Build Array (concatenate)(w533, w535) -> (w534:string[][])
        n324 = local write "Command Params"(w534) -> ()
        n325 = local write "Cmd Status"("" ("Cmd Status")) -> ()
      }
      event "Tree": Double Click {
        n326 = event-data() -> ("PlatMods"=w545:T27, "Tag"=w542:string)  [unwired: 1 in]
        n327 = Unbundle(w545) -> ("Shift"=w544:bool)  [unwired: 4 out]
        n328 = String Subset(string=w542, length (rest)=1 ("length (rest)")) -> (substring=w541:string)  [unwired: 1 in]
        n329 = Not(x=w544) -> (.not. x?=w543:bool)
        n330 = case shown="\"/\"" w541 {
          tunnel: w542 -> [_ w548]
          tunnel: w543 -> [_ w547]
          frame Default {
          }
          frame "/" {
            n331 = call <vilib>:"NT Update Persistence.vi"("Persistence"=w547, "Name"=w548) -> ()  [unwired: 9 in, 1 out]
          }
        }
      }
    }
  }
  n332 = while {
    tunnel: w91 -> [w550]
    i -> [w553]
    stop <- FALSE stop-if-true
    n333 = Wait (ms)(milliseconds to wait=u32 100) -> ()  [unwired: 1 out]
    n334 = case shown="\"Playback\"" "Rec Mode" {
      tunnel: w553 -> [_ _ w568]
      tunnel: [u32 2829099 ("Base Color") u32 11141120 ("Target Color") w557] -> w549
      frame "Stop", Default {
        # "Reset the color, extra updates don't cost much"
      }
      frame "Record" {
      }
      frame "Playback" {
        # "Playback"
        n335 = Quotient & Remainder(x=w568, y=u32 50 ("milliseconds to wait")) -> (x-y*floor(x/y)=w564:u32)  [unwired: 1 out]
        n336 = Divide(x=w564, y=u32 50 ("milliseconds to wait")) -> (x/y=w561:dbl)
        n337 = Multiply(x=6.283185307179586, y=w561) -> (x*y=w566:dbl)
        n338 = Sine(x=w566) -> (sin(x)=w565:dbl)
        n339 = Absolute Value(x=w565) -> (abs(x)=w558:dbl)
        n340 = call "Interpolate RGB Color.vi"("Proportion"=w558, "Target Color"=u32 30976, "Base Color"=u32 2829099) -> ("Result Color"=w557:u32)  [unwired: 8 in]
      }
    }
    n341 = property class="Pane"(reference=w550, "PaneColor"=w549) -> ()  [unwired: 1 in, 2 out]
  }
  n342 = local write "Dashboard Tab"(T2."Drive" ("Dashboard Tab")) -> ()
  n343 = property on="On/Off" class="Bool (strict)"("Visible"=w62) -> ()  [unwired: 2 in, 2 out]
  n344 = property on="Motor" class="Clust (strict)"("Visible"=w62) -> ()  [unwired: 2 in, 2 out]
  n345 = property on="Progress" class="Clust (strict)"("Visible"=w62) -> ()  [unwired: 2 in, 2 out]
  n346 = property on="Test Ring" class="Ring (strict)"("Visible"=w62) -> ()  [unwired: 2 in, 2 out]
  n347 = property on="Rev/Fwd" class="Clust (strict)"("Visible"=w62) -> ()  [unwired: 2 in, 2 out]
  n348 = while {
    tunnel: u16 1741 ("timeout ms (25000)") -> [w570]
    stop <- FALSE stop-if-true
    n349 = TCP Create Listener(10:w570) -> (0:w569:errorcluster, 3:w571:refnum<k5>)  [unwired: 4 in, 1 out]
    n350 = case shown="No Error" w569 {
      selector: w569 -> [w573 _]
      tunnel: w571 -> [w574 _]
      frame No Error {
        n351 = while {
          tunnel: w574 -> [w577]
          tunnel: w573 -> [w576]
          stop <- FALSE stop-if-true
          n352 = TCP Wait On Listener(8:w576, 11:w577) -> (0:w578:errorcluster, 4:w579:refnum<k5>)  [unwired: 2 in, 3 out]
          n353 = local write "TCP"(w579) -> ()
          n354 = case shown="No Error" w578 {
            frame No Error {
            }
            frame Error {
              n355 = Wait (ms)(milliseconds to wait=u32 1000) -> ()  [unwired: 1 out]
            }
          }
        }
      }
      frame Error {
        n356 = Wait (ms)(milliseconds to wait=u32 1000) -> ()  [unwired: 1 out]
      }
    }
  }
  n357 = local write "Command Selection"(u16 0 ("milliseconds to wait")) -> ()
  n358 = local write "Command Params"(string[][] [] ("Command Params")) -> ()
  n359 = global write "WPI_DashboardLogging Global.vi" "Recording"(w85) -> ()
  n360 = local write "Rec Mode"(w85) -> ()
  n361 = call <vilib>:"NT Write String.vi"("String"="Select Auto", "Name"="Auto Selector") -> ()  [unwired: 9 in, 1 out]
